vi "Clear Accurate Measure Time Out_2.vi"(6 "Sample Count (1)":i32, 7 "ESP32 ref":refnum<visa-resource-name>="COM4", 8 "error in (no error)":errorcluster, 11 "DMM ref":refnum<visa-resource-name>) -> (0 "error out":errorcluster, 1 "error?":bool, 2 "Time out count":i32, 3 "VISA Refnum out":refnum<visa-resource-name>, 4 "lost connection":bool)   [LabVIEW 2023]
uses:
  <vilib>/Utility/error.llb/DialogType.ctl
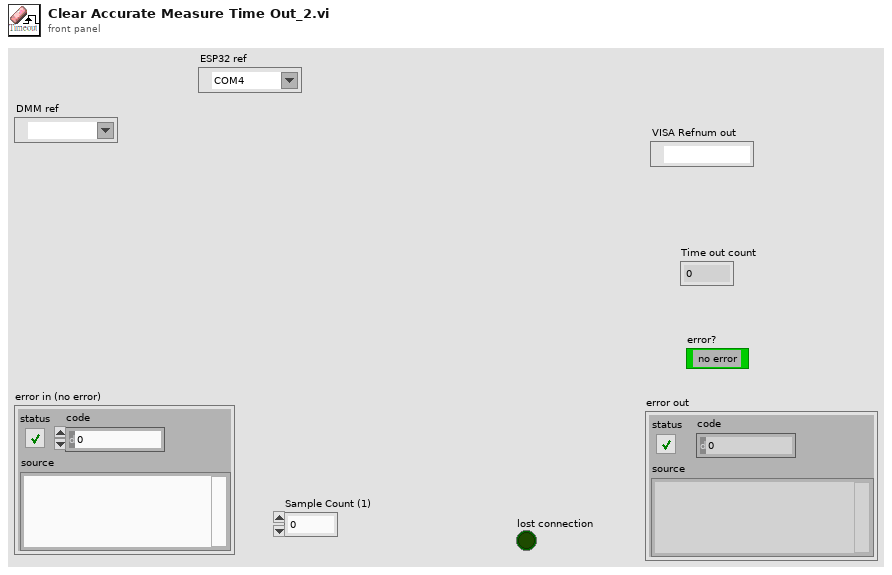
[diagram p1: front panel]
types:
  T1 = typedef "DialogType.ctl" = u16
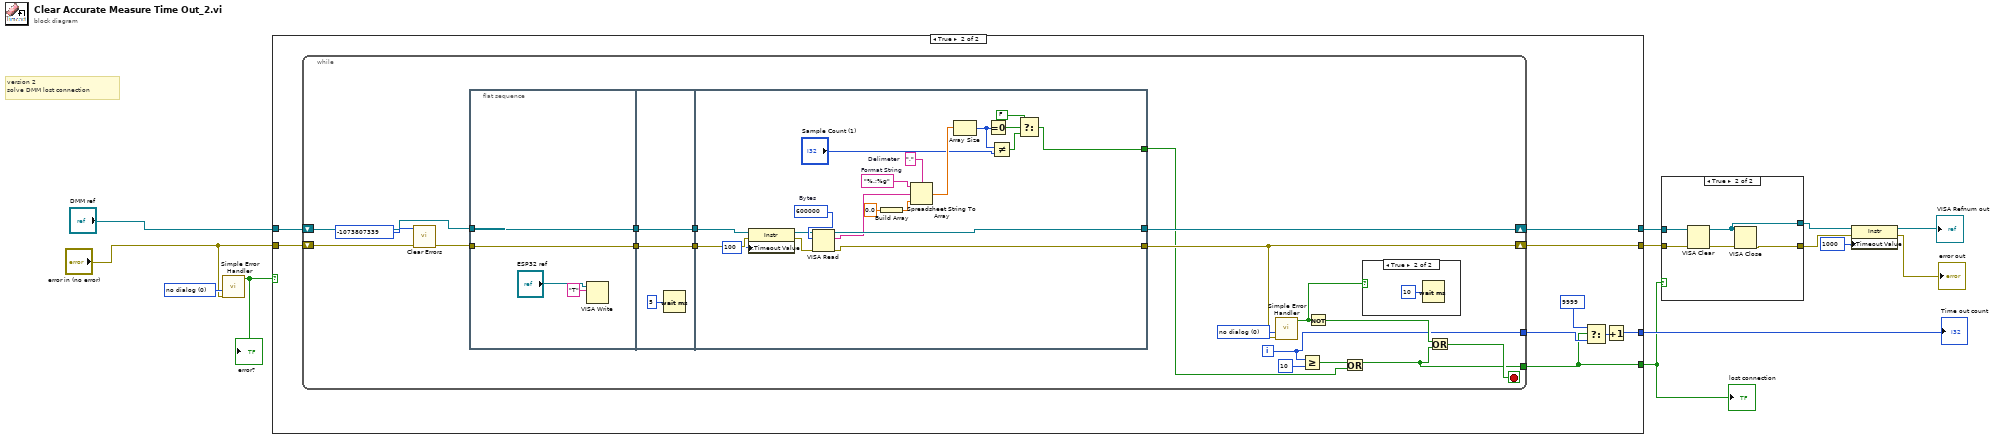
[diagram p0: block diagram]
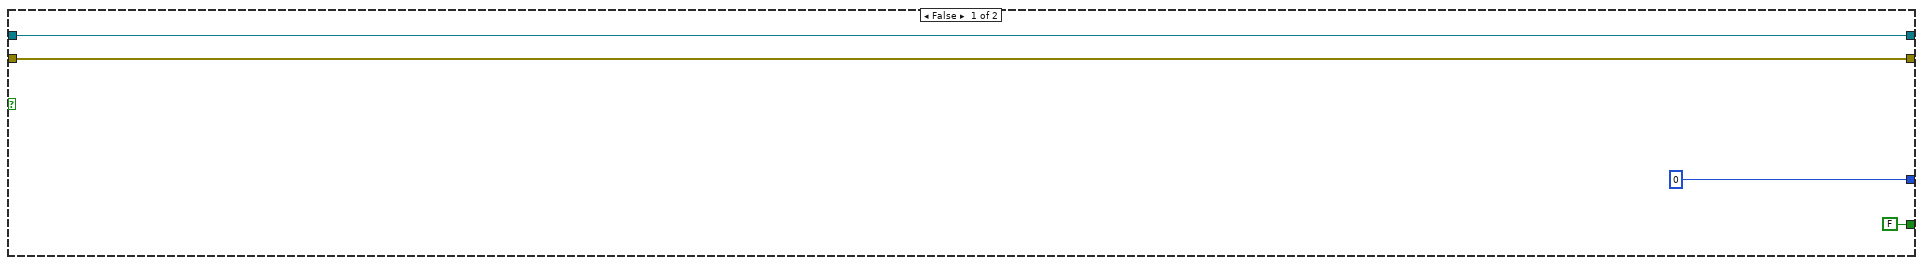
[diagram p3: hidden frame]
diagram:
  w12 = T1 0 items=["no dialog", "OK message", "continue or stop message", "OK message + warnings", "continue/stop + warnings"] ("type of dialog (OK msg:1)")
  # "version 2\nsolve DMM lost connection"
  n1 = call <vilib>:"Simple Error Handler.vi"("type of dialog (OK msg:1)"=w12, "error in (no error)"="error in (no error)") -> ("error?"=w10:bool)  [unwired: 3 in, 4 out]
  "error?" <- w10
  n2 = case shown="True" w10 {
    tunnel: [w17 w26] -> w5
    tunnel: "error in (no error)" -> [w16 w25]
    tunnel: "DMM ref" -> [w17 w24]
    tunnel: [w16 w23] -> w4
    tunnel: [0 w19] -> w9
    tunnel: [FALSE w18] -> w1
    frame False {
    }
    frame True {
      n3 = while {
        shift-right: [w39] -> w23
        shift-left: w25 -> [w43]
        shift-right: [w45] -> w26
        shift-left: w24 -> [w41]
        tunnel: [w35] -> w20
        tunnel: [w28] -> w18
        i -> [w35]
        stop <- w36 stop-if-true
        w40 = T1 0 items=["no dialog", "OK message", "continue or stop message", "OK message + warnings", "continue/stop + warnings"] ("type of dialog (OK msg:1)")
        n4 = call <vilib>:"Clear Errors.vi"("error in (no error)"=w43, "specific error code to clear (0: all)"=-1073807339 ("code out")) -> ("error out"=w42:errorcluster)  [unwired: 4 in, 1 out]
        n5 = flat-sequence {
          tunnel: w42 -> [w49]
          tunnel: w41 -> [w50]
          tunnel: [w50] -> w30
          tunnel: [w49] -> w32
          tunnel: w32 -> [w53]
          tunnel: [w53] -> w31
          tunnel: w30 -> [w52]
          tunnel: [w52] -> w29
          tunnel: [w72] -> w39
          tunnel: [w73] -> w45
          tunnel: w29 -> [w70]
          tunnel: w31 -> [w68]
          tunnel: [w54] -> w27
          frame #0 {
            n6 = VISA Write(VISA resource name="ESP32 ref", write buffer="T") -> ()  [unwired: 1 in, 3 out]
          }
          frame #1 {
            n7 = Wait (ms)(milliseconds to wait=u32 5) -> ()  [unwired: 1 out]
          }
          frame #2 {
            w64 = ","  # Delimeter
            w65 = "%.;%g"  # Format String
            w71 = u32 600000  # Bytes
            n8 = property class="Instr"(reference=w70, error in=w68, "General Settings:Timeout Value"=u32 100) -> (reference out=w69:refnum<visa-resource-name>, error out=w67:errorcluster)
            n9 = VISA Read(VISA resource name=w69, byte count=w71, error in (no error)=w67) -> (VISA resource name out=w73:refnum<visa-resource-name>, read buffer=w56:string, error out=w72:errorcluster)  [unwired: 1 out]
            n10 = Build Array(0.0) -> (w62:dbl[])
            n11 = Spreadsheet String To Array(delimiter (Tab)=w64, format string=w65, spreadsheet string=w56, array type (2D Dbl)=w62) -> (array=w61:dbl[])
            n12 = Array Size(array=w61) -> (size(s)=w57:i32)
            n13 = Equal To 0?(x=w57) -> (x = 0?=w60:bool)
            n14 = Not Equal?(x=w57, y="Sample Count (1)") -> (x != y?=w59:bool)
            n15 = Select(t=FALSE, s=w60, f=w59) -> (s? t:f=w54:bool)
          }
        }
        n16 = call <vilib>:"Simple Error Handler.vi"("type of dialog (OK msg:1)"=w40, "error in (no error)"=w39) -> ("error?"=w33:bool)  [unwired: 3 in, 4 out]
        n17 = Greater Or Equal?(x=w35, y=10) -> (x >= y?=w34:bool)
        n18 = Not(x=w33) -> (.not. x?=w37:bool)
        n19 = Or(x=w34, y=w27) -> (x .or. y?=w28:bool)
        n20 = case shown="True" w33 {
          frame False {
          }
          frame True {
            n21 = Wait (ms)(milliseconds to wait=u32 10) -> ()  [unwired: 1 out]
          }
        }
        n22 = Or(x=w37, y=w28) -> (x .or. y?=w36:bool)
      }
      n23 = Select(t=9999, s=w18, f=w20) -> (s? t:f=w21:i32)
      n24 = Increment(x=w21) -> (x+1=w19:i32)
    }
  }
  "Time out count" <- w9
  "lost connection" <- w1
  n25 = case shown="True" w1 {
    tunnel: w5 -> [w75 w79]
    tunnel: w4 -> [w74 w80]
    tunnel: [w74 w77] -> w2
    tunnel: [w75 w76] -> w3
    frame False {
    }
    frame True {
      n26 = VISA Clear(VISA resource name=w79, error in (no error)=w80) -> (VISA resource name out=w76:refnum<visa-resource-name>, error out=w78:errorcluster)
      n27 = VISA Close(VISA resource name=w76, error in (no error)=w78) -> (error out=w77:errorcluster)
    }
  }
  n28 = property class="Instr"(reference=w3, error in=w2, "General Settings:Timeout Value"=u32 1000) -> (reference out=→"VISA Refnum out":refnum<visa-resource-name>, error out=→"error out":errorcluster)
